vi "Lift_State.vi"(9 "Drive Control":T1 {"Power (100)" min=-100 max=100}, 10 "Datalog In":i32[](array[numeric]), 11 "Dump Open":u8) -> (2 "Datalog Out":i32[](array[numeric]))   [LabVIEW 2012, in "Serenity_mk2.lvrbt"]
uses:
  Serenity_mk2.lvrbt
  SubVIs/auto_drive_TYP.ctl
  <vilib>/NXT/Hardware/Plugins/Tetrix DC Motor/TetrixDCMotorAddress.ctl
  <vilib>/NXT/Hardware/Plugins/Tetrix 180 deg Servo/Tetrix180ServoAddress.ctl
  <vilib>/NXT/NXTIO Xnodes/NXTIONodeSubVIs/TETRIX IO Move DC Motors.vi
  <vilib>/NXT/Dual Mode Library/Display/drawNumber.vi
  <vilib>/NXT/NXTIO Xnodes/NXTIONodeSubVIs/TETRIX IO Motor Status.vi
  <vilib>/NXT/NXTIO Xnodes/NXTIONodeSubVIs/TETRIX IO Stop DC Motors.vi
  <vilib>/NXT/Dual Mode Library/Sound/Tone.vi
  <vilib>/NXT/NXTIO Xnodes/NXTIONodeSubVIs/TETRIX IO Move Servos.vi
  <vilib>/NXT/NXTIO Xnodes/AddressXNode/NXTIOAddress.xnode
  <vilib>/NXT/Subs/LVHSConnector.ctl
  <vilib>/NXT/NXTIO Xnodes/NXTIOXNode/NXTIO.xnode
  <vilib>/NXT/LegoClasses/BrickReference/BrickReference.lvclass
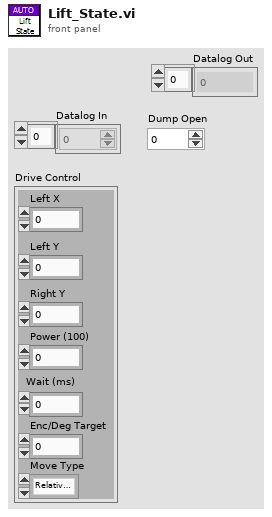
[diagram p1: front panel]
types:
  T1 = typedef "auto_drive_TYP.ctl" = cluster{"Left X":i8, "Left Y":i8, "Right Y":i8, "Power (100)":i8, "Wait (ms)":u32, "Enc/Deg Target":i32, "Move Type":enum16{"Relative Degrees", "Wait", "Encoder"}}
  T2 = typedef "TetrixDCMotorAddress.ctl" = i32
  T3 = typedef "LVHSConnector.ctl" = refnum<class "BrickReference.lvclass">
  T4 = typedef "Tetrix180ServoAddress.ctl" = i32
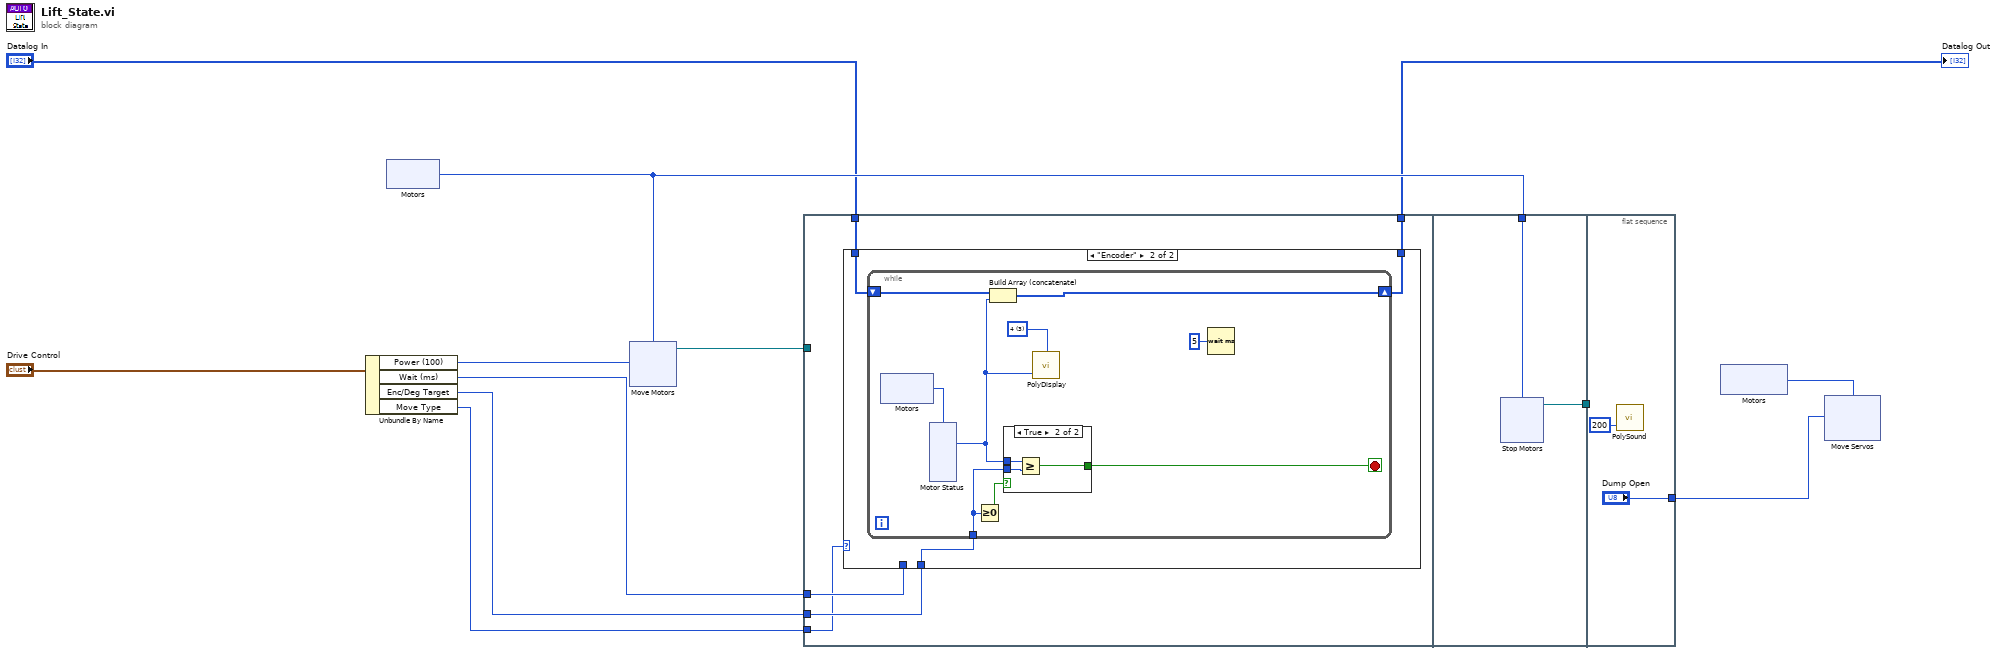
[diagram p0: block diagram]
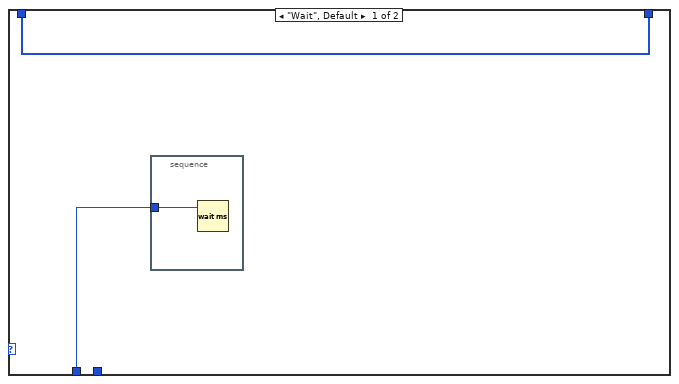
[diagram p2: hidden frame]
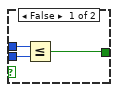
[diagram p3: hidden frame]
diagram:
  n1 = Unbundle By Name("Drive Control") -> ("Power (100)"=w9:i8, "Wait (ms)"=w6:u32, "Enc/Deg Target"=w7:i32, "Move Type"=w11:enum16{"Relative Degrees", "Wait", "Encoder"})
  n2 = xnode "Motors"() -> ("Motor"=w8:T2)
  n3 = xnode "Move Motors"("Power/Speed 1"=w9, "Motors"=w8) -> ("NXT/EV3"=w10:T3)  [unwired: 1 in]
  n4 = flat-sequence {
    tunnel: w6 -> [w17]
    tunnel: w7 -> [w16]
    tunnel: w11 -> [w15]
    tunnel: "Datalog In" -> [w14]
    tunnel: [w13] -> w5
    tunnel: w10 -> [_]
    tunnel: w8 -> [w49]
    tunnel: [w48] -> w12
    tunnel: w12 -> [_]
    tunnel: ["Dump Open"] -> w2
    frame #0 {
      n5 = case shown="\"Encoder\"" w15 {
        tunnel: w17 -> [w18 _]
        tunnel: w16 -> [_ w23]
        tunnel: w14 -> [w19 w22]
        tunnel: [w19 w21] -> w13
        frame "Wait", Default {
          n6 = stacked-sequence {
            tunnel: w18 -> [w20]
            frame #0 {
              n7 = Wait (ms)(milliseconds to wait=w20) -> ()  [unwired: 1 out]
            }
          }
        }
        frame "Encoder" {
          n8 = while {
            tunnel: w23 -> [w27]
            shift-right: [w31] -> w21
            shift-left: w22 -> [w30]
            stop <- w28 stop-if-true
            w25 = i16 3 items=["1", "2", "3", "4", "5", "6", "7", "8", "9", "10", "11", "12"] ("Line")
            n9 = xnode "Motors"() -> ("Motor"=w32:T2)
            n10 = xnode "Motor Status"("Motors"=w32) -> ("Position 1"=w26:i32)  [unwired: 1 in, 2 out]
            n11 = Greater Or Equal To 0?(x=w27) -> (x >= 0?=w29:bool)
            n12 = Build Array (concatenate)(w30, w26) -> (w31:i32[])
            n13 = case shown="True" w29 {
              tunnel: w26 -> [w35 w38]
              tunnel: [w33 w37] -> w28
              tunnel: w27 -> [w34 w36]
              frame False {
                n14 = Less Or Equal?(x=w35, y=w34) -> (x <= y?=w33:bool)
              }
              frame True {
                n15 = Greater Or Equal?(x=w38, y=w36) -> (x >= y?=w37:bool)
              }
            }
            n16 = call-poly <vilib>:"PolyDisplay.vi"("number"=w26, "Line"=w25) -> ()  [unwired: 2 in, 1 out]
            n17 = Wait (ms)(milliseconds to wait=u32 5) -> ()  [unwired: 1 out]
          }
        }
      }
    }
    frame #1 {
      n18 = xnode "Stop Motors"("Motors"=w49) -> ("NXT/EV3"=w48:T3)  [unwired: 1 in]
    }
    frame #2 {
      n19 = call-poly <vilib>:"PolySound.vi"("Duration (500 ms)"=u16 200) -> ()  [unwired: 3 in, 1 out]
    }
  }
  n20 = xnode "Motors"() -> ("Motor"=w1:T4)
  n21 = xnode "Move Servos"("Position 1"=w2, "Motors"=w1) -> ()  [unwired: 1 in, 1 out]
  "Datalog Out" <- w5
